vi "__init__.vi"(8 "error in (no error)":errorcluster, 9 "Frequency (Hz)":dbl=32768.0, 10 "Amplitude (V rms)":dbl=0.001, 11 "VISA resource name":refnum<visa-resource-name>) -> (0 "error out":errorcluster, 3 "Keysight 33511B out":refnum<class "Keysight 33511B.lvclass">)   [LabVIEW 2020, in "Keysight 33511B.lvclass"]
uses:
  Keysight 33511B.lvclass
  Keysight 33511B.lvclass/Keysight 33511B.ctl
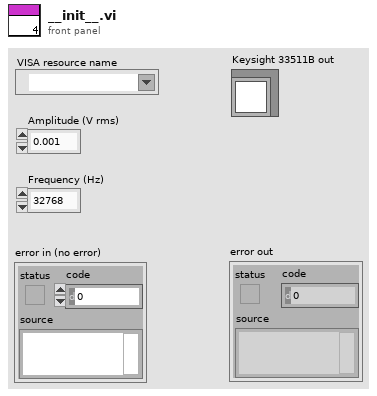
[diagram p1: front panel]
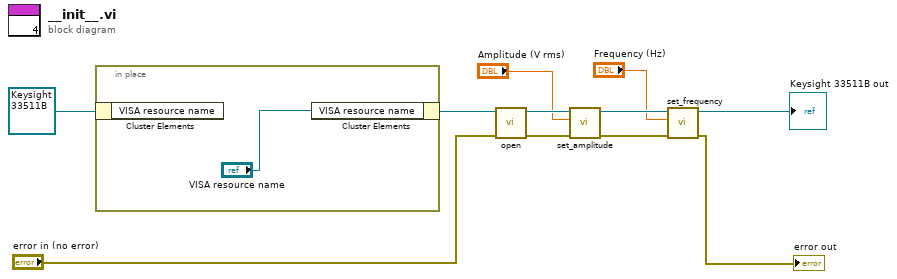
[diagram p0: block diagram]
diagram:
  n1 = in-place {
    n2 = in-place-cluster #1(refnum<class "Keysight 33511B.lvclass"> refnum ("Keysight 33511B out")) -> ()  [unwired: 1 out]
    n3 = in-place-cluster #1("VISA resource name"="VISA resource name") -> (w10:refnum<class "Keysight 33511B.lvclass">)
  }
  n4 = call-dynamic "open.vi"("error in (no error)"="error in (no error)", "Keysight 33500B in"=w10) -> ("error out"=w7:errorcluster, "Keysight 33500B out"=w8:refnum<class "Keysight 33511B.lvclass">)  [unwired: 8 in]
  n5 = call-dynamic "set_amplitude.vi"("error in (no error)"=w7, "Amplitude (Vpp)"="Amplitude (V rms)", "Keysight 33511B in"=w8) -> ("error out"=w4:errorcluster, "Keysight 33511B out"=w5:refnum<class "Keysight 33511B.lvclass">)  [unwired: 7 in]
  n6 = call-dynamic "set_frequency.vi"("error in (no error)"=w4, "Frequency"="Frequency (Hz)", "Keysight 33511B in"=w5) -> ("error out"=→"error out":errorcluster, "Keysight 33511B out"=→"Keysight 33511B out":refnum<class "Keysight 33511B.lvclass">)  [unwired: 7 in]
